vi "Read Array Control.vi"(5 "section":string, 7 "Prefix":string, 8 "Error In":errorcluster, 10 "File refnum":T1, 11 "Ctl Refnum":refnum<vi>) -> (0 "Error Out":errorcluster, 2 "File refnum out":T1, 3 "Ctl Refnum out":refnum<vi>)   [LabVIEW 2015]
uses:
  <vilib>/Utility/config.llb/Config Data RefNum.ctl
  <vilib>/Utility/Data Type/NI_Data Type.lvlib
  <vilib>/Utility/config.llb/NI_LVConfig.lvlib
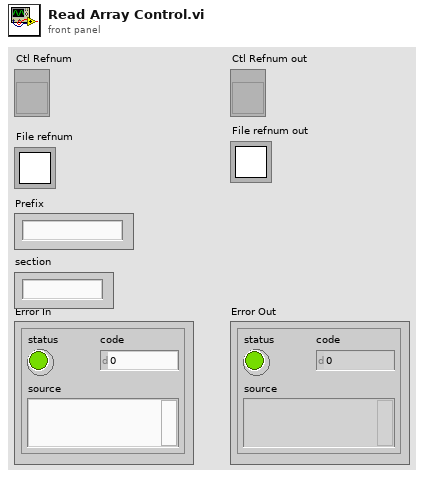
[diagram p1: front panel]
types:
  T1 = typedef "NI_LVConfig.lvlib/Config Data RefNum.ctl" = refnum<k1>
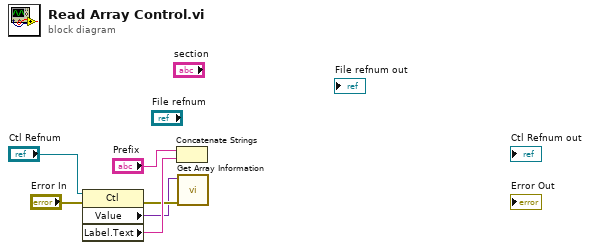
[diagram p0: block diagram]
diagram:
  n1 = property class="Ctl"(reference="Ctl Refnum", error in="Error In") -> (error out=w3:errorcluster, "Value"=w1:variant, "Label.Text"=w4:string)  [unwired: 1 out]
  n2 = Concatenate Strings("Prefix", w4) -> ()  [unwired: 1 out]
  n3 = call <vilib>:"Get Array Information.vi"("error in (no error)"=w3, "Variant"=w1) -> ()  [unwired: 6 in, 4 out]
